vi "Stream data.vi"(6 "state":string, 8 "error in (no error)":errorcluster, 11 "Data":T1={"link 1 angle"=0.0, "link 2 angle"=0.0, "link 1 length"=0.0, "link 2 length"=0.0, "Current arm location"=[{"X"=0.0, "Y"=0.0}, {"X"=-37.249783598972314, "Y"=33.353464914904016}, {"X"=-74.49956719794463, "Y"=66.70692982980803}], "Link Picture"=bytes[1162], "Desired Location"={"Desired X"=0.0, "Desired Y"=0.0}, "Next Location"={"Next X"=0.0, "Next Y"=0.0}, "Error"={"Joint1 error"=0.0, "Joint2 error"=0.0}, "tdms data"=refnum, "de/dt"={"joint1 de/dt"=0.0, "joint2 de/dt"=0.0}, "Voltages"={"Joint1 voltage"=0.0, "Joint2 voltage"=0.0}, "Time"=0.0, "dt"=0.0, "counts/rev"=0.0, "kp"=0.0, "kd"=0.0, "ki"=0.0, "Int(error)"={"joint1 int(e)"=0.0, "joint2 int(e)"=0.0}, "Desired angles"={"theta 1"=0.0, "theta 2"=0.0}, "Current counts"={"theta 1"=0.0, "theta 2"=0.0}, "Desired Counts"={"theta 1"=0.0, "theta 2"=0.0}, "Preivous Error"={"Joint1 Previous error"=0.0, "Joint2 Previous error"=0.0}, "Counts/s"=0.0, "Correct counter"=0}) -> (0 "error out":errorcluster, 3 "tdms file out":refnum<k34>)   [LabVIEW 2017]
uses:
  Type Defs/Host Data.ctl
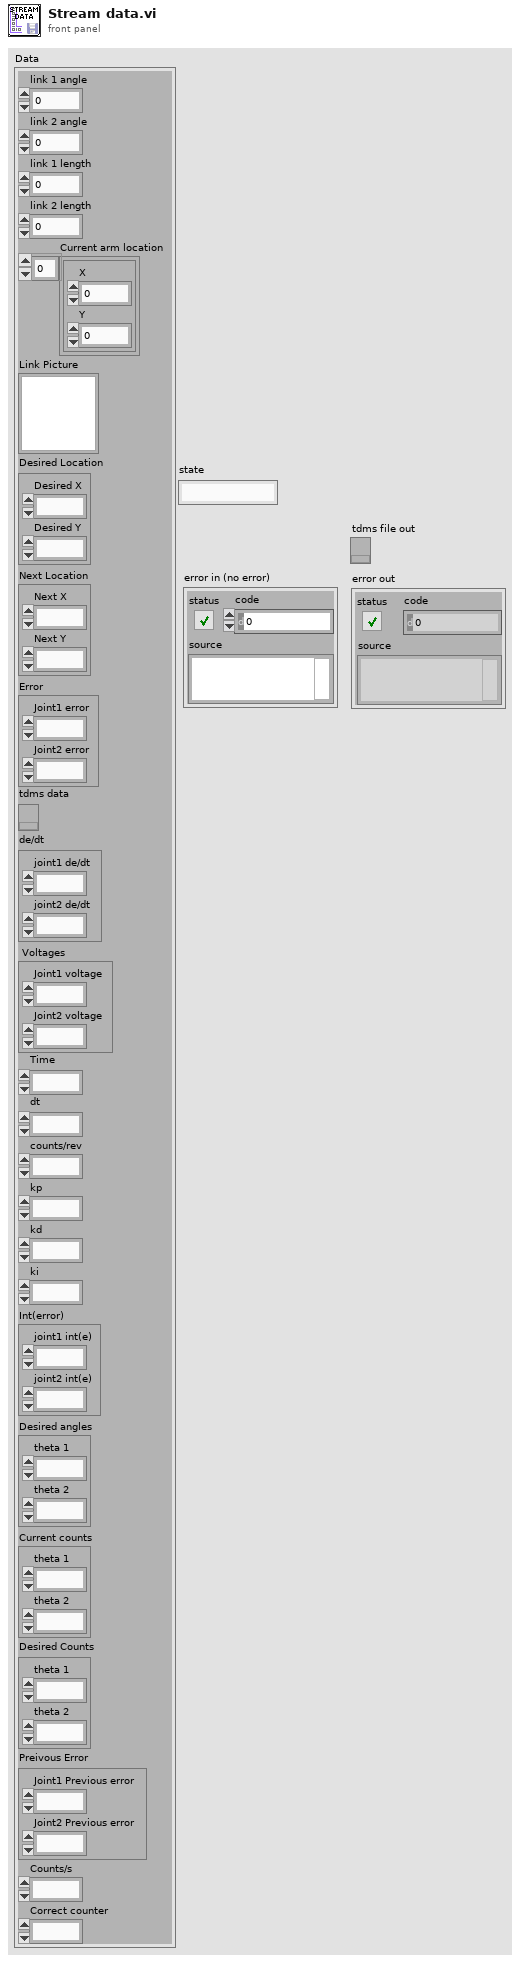
[diagram p1: front panel]
types:
  T1 = typedef "Host Data.ctl" = cluster{"link 1 angle":dbl, "link 2 angle":dbl, "link 1 length":dbl, "link 2 length":dbl, "Current arm location":cluster{"X":dbl, "Y":dbl}[], "Link Picture":picture, "Desired Location":cluster{"Desired X":dbl, "Desired Y":dbl}, "Next Location":cluster{"Next X":dbl, "Next Y":dbl}, "Error":cluster{"Joint1 error":dbl, "Joint2 error":dbl}, "tdms data":refnum<k34>, "de/dt":cluster{"joint1 de/dt":dbl, "joint2 de/dt":dbl}, "Voltages":cluster{"Joint1 voltage":dbl, "Joint2 voltage":dbl}, "Time":dbl, "dt":dbl, "counts/rev":dbl, "kp":dbl, "kd":dbl, "ki":dbl, "Int(error)":cluster{"joint1 int(e)":dbl, "joint2 int(e)":dbl}, "Desired angles":cluster{"theta 1":dbl, "theta 2":dbl}, "Current counts":cluster{"theta 1":dbl, "theta 2":dbl}, "Desired Counts":cluster{"theta 1":dbl, "theta 2":dbl}, "Preivous Error":cluster{"Joint1 Previous error":dbl, "Joint2 Previous error":dbl}, "Counts/s":dbl, "Correct counter":i32}
  T2 = cluster{"Joint1 voltage":dbl, "Joint2 voltage":dbl}
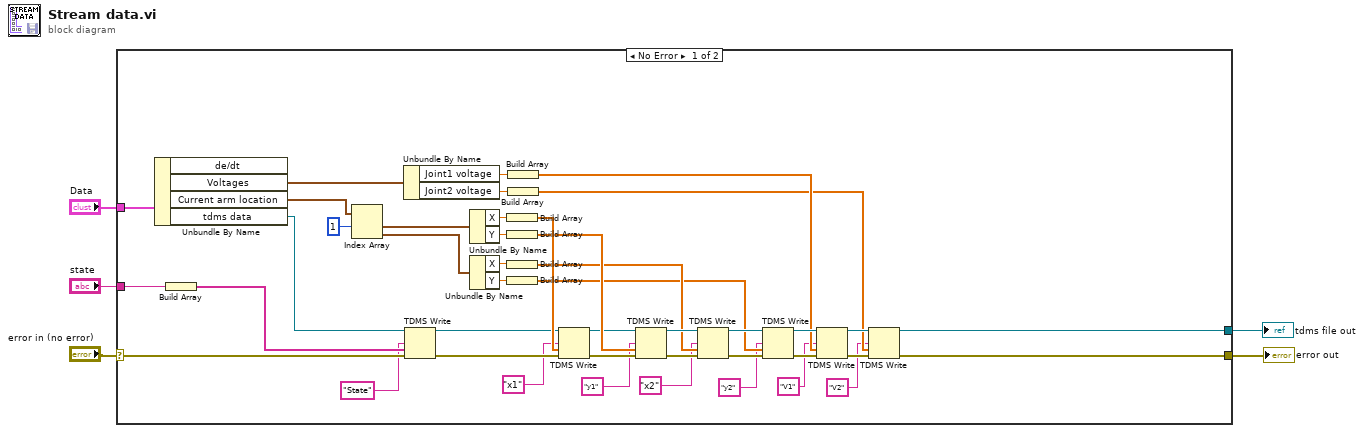
[diagram p0: block diagram]
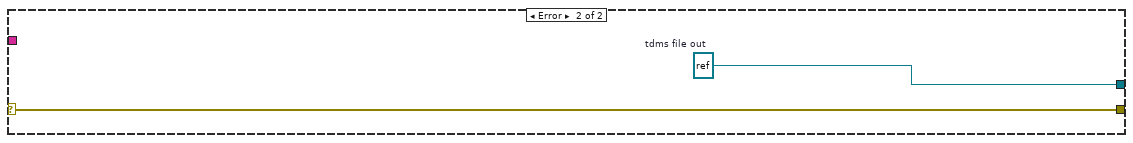
[diagram p2: hidden frame]
diagram:
  n1 = case shown="No Error" "error in (no error)" {
    selector: "error in (no error)" -> [w31 w50]
    tunnel: "Data" -> [w48 _]
    tunnel: [w6 w50] -> w3
    tunnel: "state" -> [w27 _]
    tunnel: [w7 w49] -> w1
    frame No Error {
      n2 = Unbundle By Name(w48) -> ("Voltages"=w18:T2, "Current arm location"=w47:cluster{"X":dbl, "Y":dbl}[], "tdms data"=w35:refnum<k34>)  [unwired: 1 out]
      n3 = Build Array(w27) -> (w26:string[])
      n4 = Index Array(array=w47, index #1=1) -> (element #1=w46:cluster{"X":dbl, "Y":dbl}, element #2=w44:cluster{"X":dbl, "Y":dbl})  [unwired: 1 in]
      n5 = Unbundle By Name(w18) -> ("Joint1 voltage"=w17:dbl, "Joint2 voltage"=w16:dbl)
      n6 = TDMS Write(0:w35, 7:"State" ("group name in (Untitled)"), 9:w26, 11:w31) -> (4:w34:refnum<k34>, 15:w30:errorcluster)  [unwired: 2 in, 2 out]
      n7 = Unbundle By Name(w46) -> ("X"=w43:dbl, "Y"=w40:dbl)
      n8 = Unbundle By Name(w44) -> ("X"=w37:dbl, "Y"=w36:dbl)
      n9 = Build Array(w43) -> (w42:dbl[])
      n10 = Build Array(w40) -> (w39:dbl[])
      n11 = Build Array(w37) -> (w25:dbl[])
      n12 = Build Array(w36) -> (w24:dbl[])
      n13 = Build Array(w17) -> (w11:dbl[])
      n14 = Build Array(w16) -> (w10:dbl[])
      n15 = TDMS Write(0:w34, 7:"x1" ("group name in (Untitled)"), 9:w42, 11:w30) -> (4:w38:refnum<k34>, 15:w41:errorcluster)  [unwired: 2 in, 2 out]
      n16 = TDMS Write(0:w38, 7:"y1" ("group name in (Untitled)"), 9:w39, 11:w41) -> (4:w33:refnum<k34>, 15:w29:errorcluster)  [unwired: 2 in, 2 out]
      n17 = TDMS Write(0:w33, 7:"x2" ("group name in (Untitled)"), 9:w25, 11:w29) -> (4:w32:refnum<k34>, 15:w28:errorcluster)  [unwired: 2 in, 2 out]
      n18 = TDMS Write(0:w32, 7:"y2" ("group name in (Untitled)"), 9:w24, 11:w28) -> (4:w15:refnum<k34>, 15:w14:errorcluster)  [unwired: 2 in, 2 out]
      n19 = TDMS Write(0:w15, 7:"V1" ("group name in (Untitled)"), 9:w11, 11:w14) -> (4:w12:refnum<k34>, 15:w13:errorcluster)  [unwired: 2 in, 2 out]
      n20 = TDMS Write(0:w12, 7:"V2" ("group name in (Untitled)"), 9:w10, 11:w13) -> (4:w7:refnum<k34>, 15:w6:errorcluster)  [unwired: 2 in, 2 out]
    }
    frame Error {
      w49 = refnum<k34> refnum  # tdms file out
    }
  }
  "error out" <- w3
  "tdms file out" <- w1
